vi "Tunnel_Wiring_Wizard_LV8OK.vi"() -> ()   [LabVIEW 2010]
doc: "This utility will automatically create a wire for each case to connect two selected tunnels in a case selector or event structure.\n\nCreated by David Boyd\n02/04/2006 Modified for LV8 by Stanislav Rumega, H Vew Labs (labhsm.com)"
panel:
  out "Active VI":string
  in  "I Like to Watch":bool
  in  "Wire It!":bool
  out "Status":string
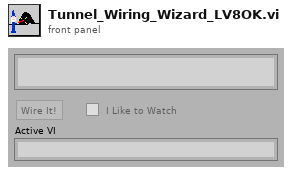
[diagram p1: front panel]
types:
  T1 = enum32{"Invalid", "Standard", "Closed", "Hidden", "Minimized", "Maximized"}
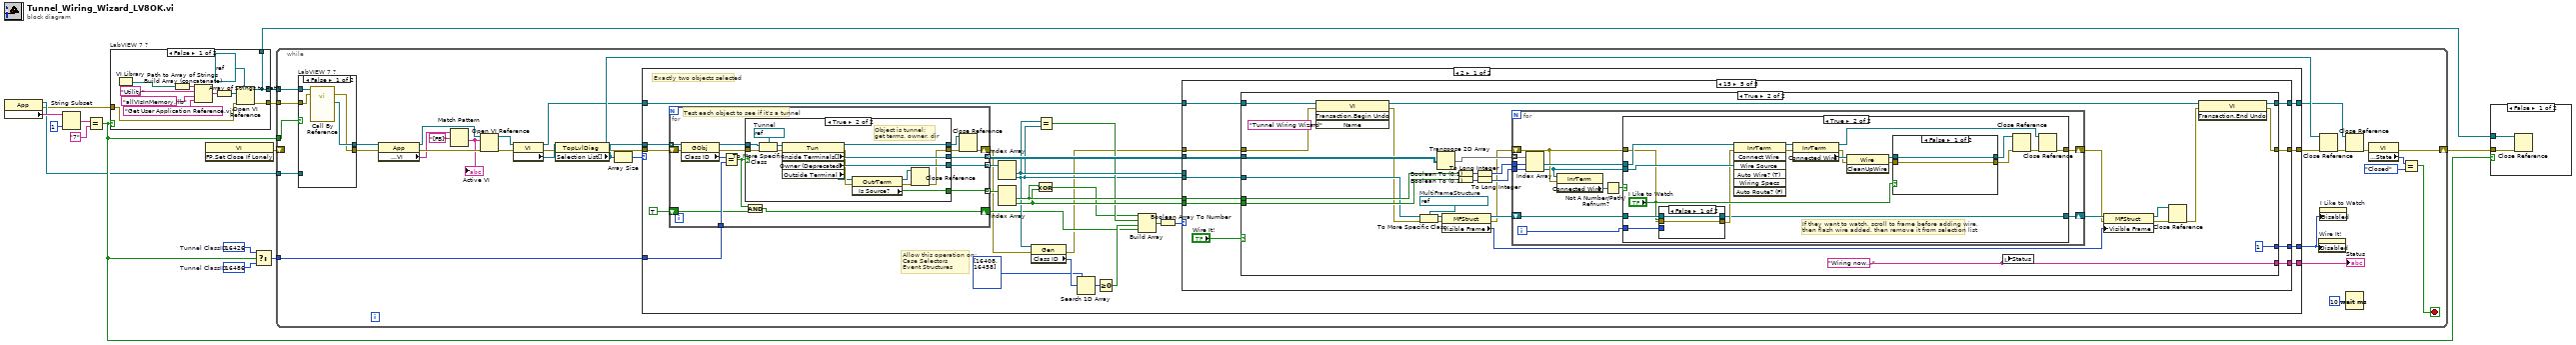
[diagram p0: block diagram]
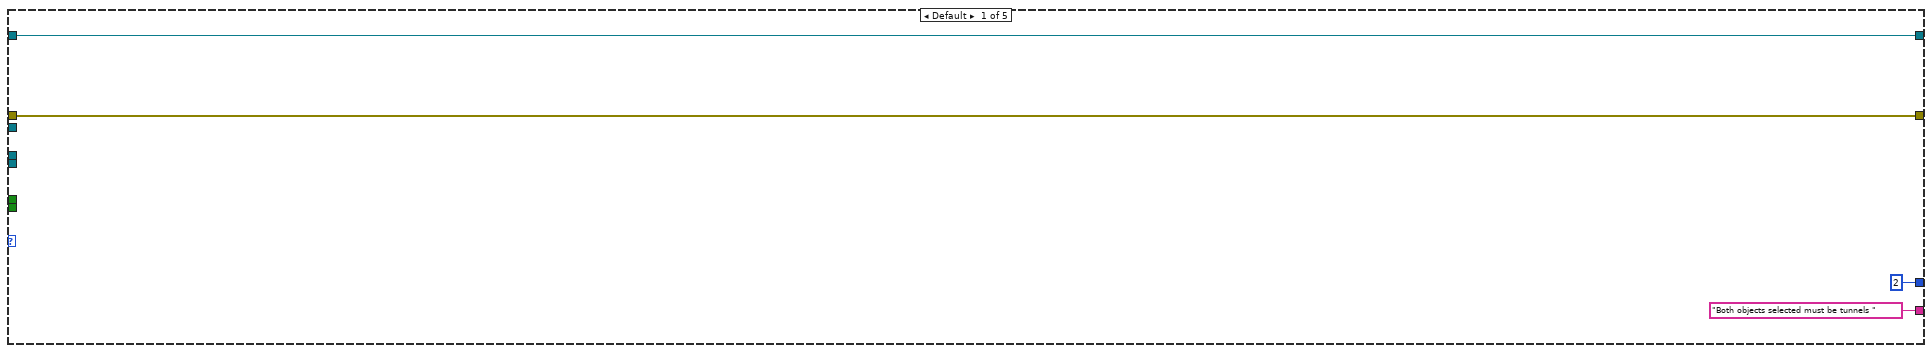
[diagram p5: hidden frame]
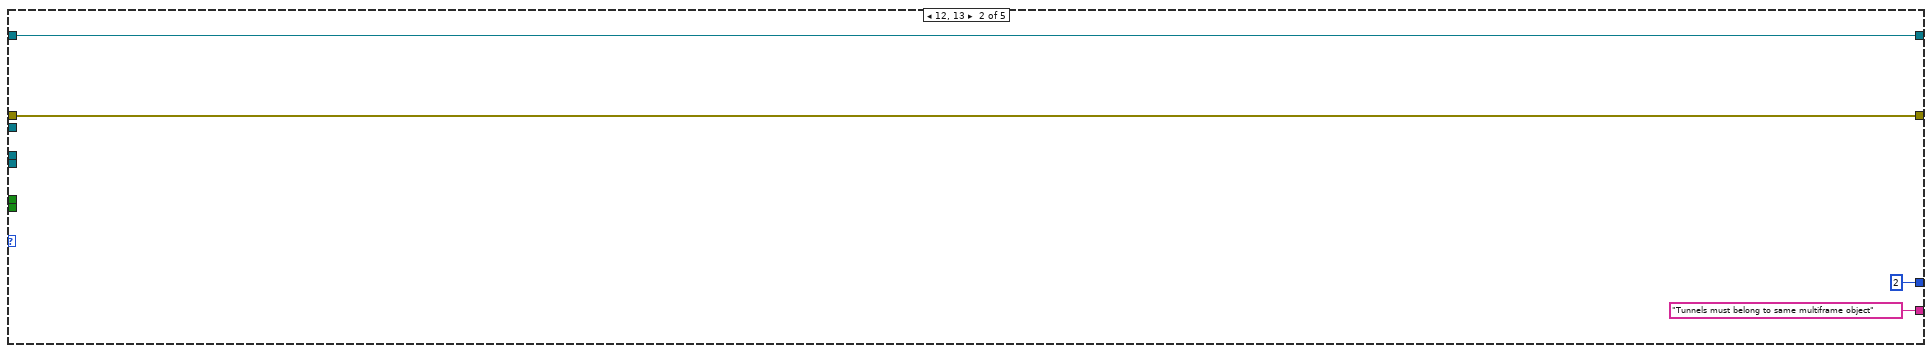
[diagram p6: hidden frame]
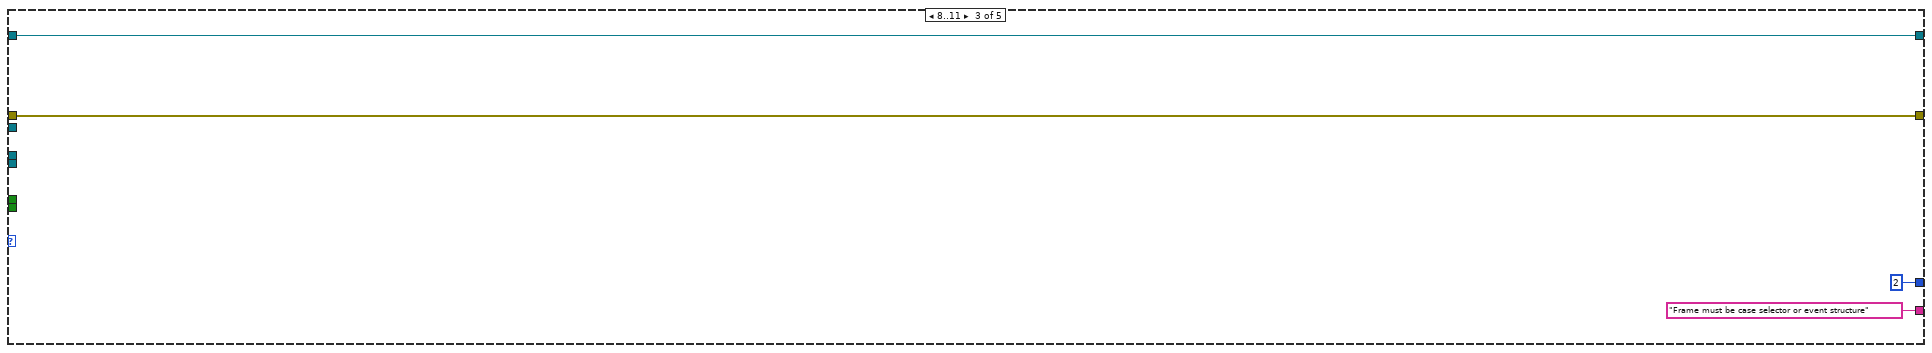
[diagram p7: hidden frame]
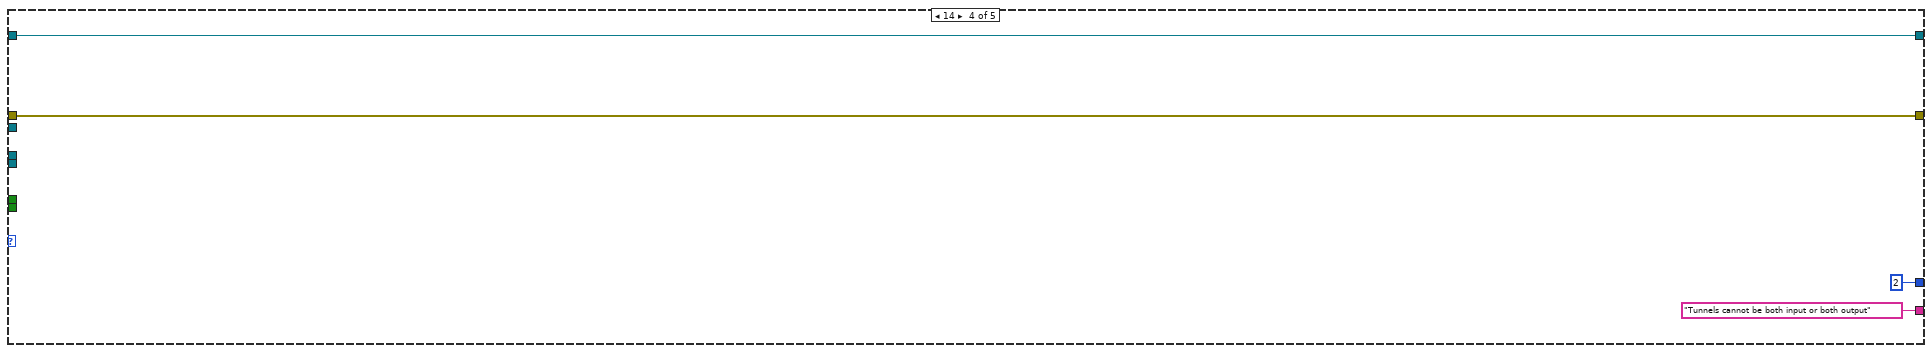
[diagram p8: hidden frame]
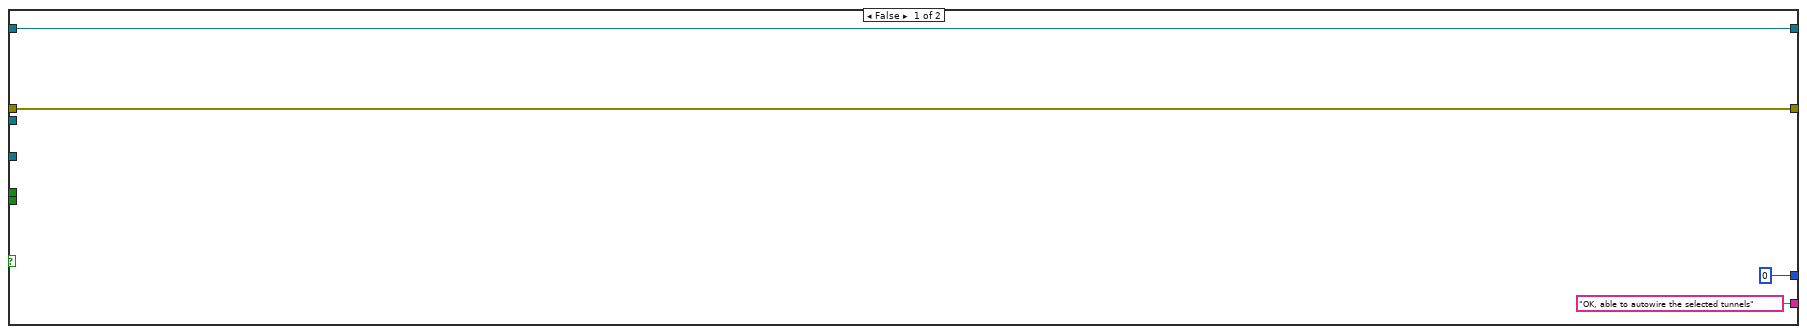
[diagram p9: hidden frame]
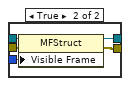
[diagram p11: hidden frame]
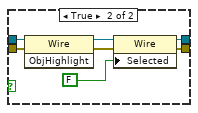
[diagram p12: hidden frame]
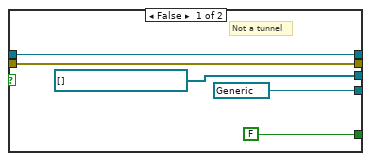
[diagram p13: hidden frame]
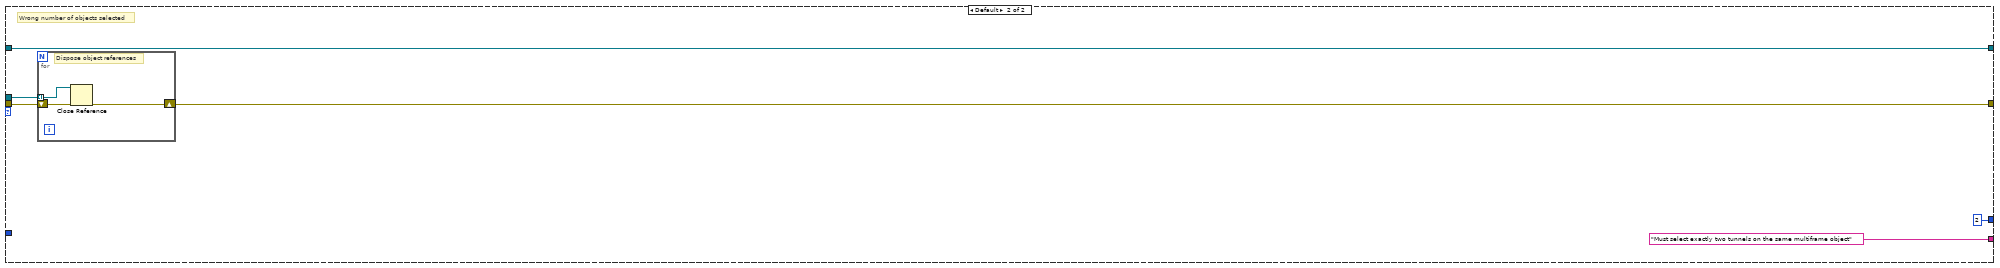
[diagram p14: hidden frame]
diagram:
  w10 = u32 16486  # Tunnel ClassID
  w11 = u32 16426  # Tunnel ClassID
  n1 = property class="App"() -> (reference out=w3:refnum<vi>, error out=w1:errorcluster, "Application:Version Number"=w15:string)  [unwired: 2 in]
  n2 = String Subset(string=w15, length (rest)=1 ("length (rest)")) -> (substring=w13:string)  [unwired: 1 in]
  n3 = Equal?(x=w13, y="7") -> (x = y?=w5:bool)
  n4 = case "LabVIEW 7 ?" shown="False" w5 {
    tunnel: [w18 _] -> w6
    tunnel: [w18 _] -> w4
    tunnel: [w17 w27] -> w2
    tunnel: w1 -> [w16 w27]
    frame False {
      n5 = VI Library() -> (path=w20:path)
      n6 = Path to Array of Strings(0:w20) -> (2:w21:string[])  [unwired: 1 out]
      n7 = Build Array (concatenate)(w21, "Utility", "allVIsInMemory.llb", "Get User Application Reference.vi") -> (w22:string[])
      n8 = Array of Strings to Path(0:w22) -> (2:w19:path)  [unwired: 1 in]
      n9 = Open VI Reference(type specifier VI Refnum (for type only)=refnum<vi> refnum, vi path=w19, error in (no error)=w16) -> (vi reference=w18:refnum<vi>, error out=w17:errorcluster)  [unwired: 3 in]
    }
    frame True {
    }
  }
  n10 = invoke class="VI" method="FP.Set Close If Lonely"() -> (error out=w8:errorcluster)  [unwired: 3 in, 2 out]
  n11 = Select(t=w11, s=w5, f=w10) -> (s? t:f=w9:u32)
  n12 = while {
    shift-right: [w39] -> w7
    shift-left: w8 -> [_]
    tunnel: w9 -> [w35]
    tunnel: w5 -> [w33]
    tunnel: w4 -> [w32]
    tunnel: w3 -> [w31]
    tunnel: w2 -> [w28]
    stop <- w36 stop-if-true
    n13 = case "LabVIEW 7 ?" shown="False" w33 {
      tunnel: w32 -> [w63 _]
      tunnel: w31 -> [_ w65]
      tunnel: [w62 w65] -> w30
      tunnel: [w61 w64] -> w29
      tunnel: w28 -> [w60 w64]
      frame False {
        n14 = call-by-ref "?"(reference=w63, error in=w60) -> (error out=w61:errorcluster, "App Refnum"=w62:refnum<vi>)  [unwired: 6 in, 2 out]
      }
      frame True {
      }
    }
    n15 = property class="App"(reference=w30, error in=w29) -> (reference out=w34:refnum<vi>, error out=w51:errorcluster, "Application:Active:VI"=w45:string)
    n16 = Match Pattern(string=w45, regular expression="[FB]") -> (after substring=w44:string)  [unwired: 1 in, 3 out]
    "Active VI" <- w44
    n17 = Open VI Reference(application reference (local)=w34, vi path=w44, error in (no error)=w51) -> (vi reference=w50:refnum<vi>, error out=w49:errorcluster)  [unwired: 3 in]
    n18 = property class="VI"(reference=w50, error in=w49) -> (reference out=w42:refnum<vi>, error out=w47:errorcluster, "Block Diagram"=w48:refnum<vi>)
    n19 = property class="TopLvlDiag"(reference=w48, error in=w47) -> (reference out=w57:refnum<vi>, error out=w59:errorcluster, "Selection List[]"=w55:refnum<vi>[])
    n20 = Array Size(array=w55) -> (size(s)=w54:i32)
    n21 = case shown="2" w54 {
      tunnel: w59 -> [w92 w241]
      tunnel: [w89 w240] -> w56
      tunnel: w55 -> [w91 w239]
      tunnel: [w84 "Must select exactly two tunnels on the same multiframe object"] -> w53
      tunnel: [w83 2] -> w52
      tunnel: w42 -> [w68 w236]
      tunnel: [w67 w236] -> w41
      tunnel: w35 -> [w66 _]
      frame 2 {
        # "Allow this operation on:\nCase Selectors\nEvent Structures"
        # "Exactly two objects selected"
        n22 = for {
          tunnel: w91 -> [w216] mode=indexing
          shift-right: [w214] -> w70
          shift-left: w92 -> [w215]
          tunnel: [w209] -> w88 mode=indexing
          tunnel: [w208] -> w85 mode=indexing
          tunnel: [w207] -> w90 mode=indexing
          tunnel: w66 -> [w205]
          shift-right: [w202] -> w71
          shift-left: TRUE -> [w204]
          # "Test each object to see if it's a tunnel"
          n23 = property class="GObj"(reference=w216, error in=w215) -> (reference out=w213:refnum<vi>, error out=w211:errorcluster, "Class ID"=w206:u32)
          n24 = Equal?(x=w206, y=w205) -> (x = y?=w203:bool)
          n25 = case shown="True" w203 {
            tunnel: w213 -> [w221 w235]
            tunnel: [w221 w231] -> w212
            tunnel: w211 -> [w220 w234]
            tunnel: [w220 w223] -> w210
            tunnel: [FALSE ("IsSource") w230] -> w209
            tunnel: [refnum<vi> refnum ("Owner") w227] -> w207
            tunnel: [refnum<vi>[] [] w228] -> w208
            frame False {
              # "Not a tunnel"
            }
            frame True {
              w233 = refnum<vi> refnum  # Tunnel
              # "Object is tunnel;\nget terms, owner, dir"
              n26 = To More Specific Class(target class=w233, reference=w235, error in=w234) -> (specific class reference=w232:refnum<vi>, error out=w229:errorcluster)
              n27 = property class="Tun"(reference=w232, error in=w229) -> (reference out=w231:refnum<vi>, error out=w224:errorcluster, "Inside Terminals[]"=w228:refnum<vi>[], "Owner (Deprecated)"=w227:refnum<vi>, "Outside Terminal"=w222:refnum<vi>)
              n28 = property class="OutrTerm"(reference=w222, error in=w224) -> (reference out=w225:refnum<vi>, error out=w226:errorcluster, "Is Source?"=w230:bool)
              n29 = Close Reference(reference=w225, error in (no error)=w226) -> (error out=w223:errorcluster)
            }
          }
          n30 = And(x=w203, y=w204) -> (x .and. y?=w202:bool)
          n31 = Close Reference(reference=w212, error in (no error)=w210) -> (error out=w214:errorcluster)
        }
        n32 = Index Array(array=w90) -> (element #1=w82:refnum<vi>, element #2=w76:refnum<vi>)  [unwired: 2 in]
        n33 = Index Array(array=w88) -> (element #1=w87:bool, element #2=w86:bool)  [unwired: 2 in]
        n34 = property class="Gen"(reference=w76, error in=w70) -> (error out=w69:errorcluster, "Class ID"=w75:u32)  [unwired: 1 out]
        n35 = Exclusive Or(1:w86, 2:w87) -> (0:w77:bool)
        n36 = Equal?(x=w82, y=w76) -> (x = y?=w78:bool)
        n37 = Search 1D Array(1D array=u32[] [16408, 16458], element=w75) -> (index of element=w73:i32)  [unwired: 1 in]
        n38 = Greater Or Equal To 0?(x=w73) -> (x >= 0?=w72:bool)
        n39 = Build Array(w77, w78, w72, w71) -> (w81:bool[])
        n40 = Boolean Array To Number(Boolean array=w81) -> (number=w80:u32)
        n41 = case shown="15" w80 {
          tunnel: [w94 w98 w103 w106 w112] -> w89
          tunnel: w87 -> [_ _ _ _ w119]
          tunnel: w86 -> [_ _ _ _ w118]
          tunnel: w85 -> [_ _ _ _ w117]
          tunnel: ["Both objects selected must be tunnels " "Tunnels must belong to same multiframe object" "Frame must be case selector or event structure" "Tunnels cannot be both input or both output" w115] -> w84
          tunnel: [2 2 2 2 w114] -> w83
          tunnel: w69 -> [w94 w98 w103 w106 w113]
          tunnel: w76 -> [_ _ _ _ w111]
          tunnel: w82 -> [_ _ _ _ _]
          tunnel: w68 -> [w93 w97 w101 w105 w110]
          tunnel: [w93 w97 w101 w105 w109] -> w67
          frame Default {
          }
          frame 12, 13 {
          }
          frame 8..11 {
          }
          frame 14 {
          }
          frame 15 {
            n42 = case shown="True" "Wire It!" {
              tunnel: w111 -> [_ w135]
              tunnel: w119 -> [_ w151]
              tunnel: w118 -> [_ w150]
              tunnel: w117 -> [_ w145]
              tunnel: ["OK, able to autowire the selected tunnels" w124] -> w115
              tunnel: [0 1] -> w114
              tunnel: w113 -> [w121 w133]
              tunnel: [w121 w131] -> w112
              tunnel: w110 -> [w120 w130]
              tunnel: [w120 w129] -> w109
              frame False {
              }
              frame True {
                w124 = "Wiring now..."
                w152 = refnum<vi> refnum  # MultiFrameStructure
                n43 = invoke class="VI" method="Transaction.Begin Undo"(reference=w130, error in=w133, "Name"="Tunnel Wiring Wizard") -> (reference out=w134:refnum<vi>, error out=w132:errorcluster)  [unwired: 1 in, 2 out]
                n44 = To More Specific Class(target class=w152, reference=w135, error in=w132) -> (specific class reference=w143:refnum<vi>, error out=w138:errorcluster)
                n45 = Transpose 2D Array(2D array=w145) -> (transposed array=w144:refnum<vi>[][])
                n46 = property class="MFStruct"(reference=w143, error in=w138) -> (reference out=w142:refnum<vi>, error out=w137:errorcluster, "Visible Frame"=w140:u32)
                n47 = Boolean To (0,1)(Boolean=w151) -> (0, 1=w149:i16)
                n48 = Boolean To (0,1)(Boolean=w150) -> (0, 1=w148:i16)
                n49 = To Long Integer(number=w149) -> (32bit integer=w147:i32)
                n50 = To Long Integer(number=w148) -> (32bit integer=w146:i32)
                n51 = for {
                  tunnel: w144 -> [w164] mode=indexing
                  shift-right: [w163] -> w136
                  shift-left: w137 -> [w159]
                  tunnel: w147 -> [w162]
                  tunnel: w146 -> [w161]
                  shift-right: [w157] -> w141
                  shift-left: w142 -> [w155]
                  i -> [w156]
                  n52 = Index Array(array=w164, index #1=w162, index #2=w161) -> (element #1=w160:refnum<vi>, element #2=w153:refnum<vi>)
                  n53 = property class="InrTerm"(reference=w153, error in=w159) -> ("Connected Wire"=w154:refnum<vi>)  [unwired: 2 out]
                  n54 = Not A Number/Path/Refnum?(number/path/refnum=w154) -> (NaN/Path/Refnum?=w158:bool)
                  n55 = case shown="True" w158 {
                    tunnel: [w166 w176] -> w163
                    tunnel: w153 -> [_ w185]
                    tunnel: w160 -> [_ w184]
                    tunnel: w159 -> [w166 w169]
                    tunnel: w155 -> [w165 w171]
                    tunnel: [w165 w167] -> w157
                    tunnel: w156 -> [_ w172]
                    frame False {
                      # "Don't add a wire to cases which already have one on the sink tunnel"
                    }
                    frame True {
                      # "If they want to watch, scroll to frame before adding wire,\nthen flash wire added, then remove it from selection list"
                      n56 = case shown="False" "I Like to Watch" {
                        tunnel: w172 -> [_ w192]
                        tunnel: w171 -> [w187 w191]
                        tunnel: [w187 w190] -> w167
                        tunnel: w169 -> [w186 w189]
                        tunnel: [w186 w188] -> w168
                        frame False {
                        }
                        frame True {
                          n57 = property class="MFStruct"(reference=w191, error in=w189, "Visible Frame"=w192) -> (reference out=w190:refnum<vi>, error out=w188:errorcluster)
                        }
                      }
                      n58 = invoke class="InrTerm" method="Connect Wire"(reference=w184, error in=w168, "Wire Source"=w185) -> (reference out=w183:refnum<vi>, error out=w182:errorcluster)  [unwired: 4 in, 5 out]
                      n59 = property class="InrTerm"(reference=w183, error in=w182) -> (reference out=w173:refnum<vi>, error out=w179:errorcluster, "Connected Wire"=w181:refnum<vi>)
                      n60 = invoke class="Wire" method="CleanUpWire"(reference=w181, error in=w179) -> (reference out=w180:refnum<vi>, error out=w178:errorcluster)  [unwired: 1 in, 1 out]
                      n61 = case shown="False" "I Like to Watch" {
                        tunnel: w178 -> [w194 w195]
                        tunnel: [w194 w196] -> w175
                        tunnel: w180 -> [w193 w198]
                        tunnel: [w193 w197] -> w174
                        frame False {
                        }
                        frame True {
                          n62 = invoke class="Wire" method="ObjHighlight"(reference=w198, error in=w195) -> (reference out=w200:refnum<vi>, error out=w201:errorcluster)  [unwired: 1 in, 1 out]
                          n63 = property class="Wire"(reference=w200, error in=w201, "Selected"=FALSE) -> (reference out=w197:refnum<vi>, error out=w196:errorcluster)
                        }
                      }
                      n64 = Close Reference(reference=w174, error in (no error)=w175) -> (error out=w177:errorcluster)
                      n65 = Close Reference(reference=w173, error in (no error)=w177) -> (error out=w176:errorcluster)
                    }
                  }
                }
                n66 = local write "Status"(w124) -> ()
                n67 = property class="MFStruct"(reference=w141, error in=w136, "Visible Frame"=w140) -> (reference out=w125:refnum<vi>, error out=w127:errorcluster)
                n68 = Close Reference(reference=w125, error in (no error)=w127) -> (error out=w126:errorcluster)
                n69 = invoke class="VI" method="Transaction.End Undo"(reference=w134, error in=w126) -> (reference out=w129:refnum<vi>, error out=w131:errorcluster)  [unwired: 1 in, 1 out]
              }
            }
          }
        }
      }
      frame Default {
        # "Wrong number of objects selected"
        n70 = for {
          tunnel: w239 -> [w243] mode=indexing
          shift-right: [w244] -> w240
          shift-left: w241 -> [w242]
          # "Dispose object references"
          n71 = Close Reference(reference=w243, error in (no error)=w242) -> (error out=w244:errorcluster)
        }
      }
    }
    "Status" <- w53
    n72 = property on="Wire It!" class="Bool"("Disabled"=w52) -> ()  [unwired: 2 in, 2 out]
    n73 = Close Reference(reference=w57, error in (no error)=w56) -> (error out=w46:errorcluster)
    n74 = property on="I Like to Watch" class="Bool (strict)"("Disabled"=w52) -> ()  [unwired: 2 in, 2 out]
    n75 = Close Reference(reference=w41, error in (no error)=w46) -> (error out=w40:errorcluster)
    n76 = Wait (ms)(milliseconds to wait=u32 10) -> ()  [unwired: 1 out]
    n77 = property class="VI"(error in=w40) -> (error out=w39:errorcluster, "Front Panel Window:State"=w38:T1)  [unwired: 1 in, 1 out]
    n78 = Equal?(x=w38, y=T1."Closed" ("Front Panel Window:State")) -> (x = y?=w36:bool)
  }
  n79 = case shown="False" w5 {
    tunnel: w7 -> [w246 _]
    tunnel: w6 -> [w245 _]
    frame False {
      n80 = Close Reference(reference=w245, error in (no error)=w246) -> ()  [unwired: 1 out]
    }
    frame True {
    }
  }
